vi "PulseLengthen.vi"(7 "Lengthen":u32, 10 "Pulse":bool) -> (2 "Lengthened":bool)   [LabVIEW 2014]
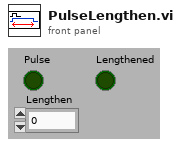
[diagram p1: front panel]
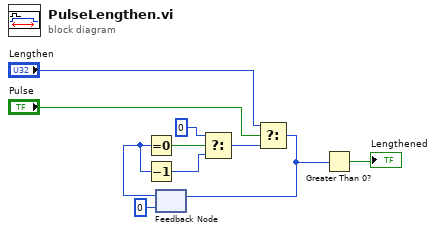
[diagram p0: block diagram]
diagram:
  n1 = feedback #1(u32 0 ("t")) -> (w2:u32)
  n2 = Equal To 0?(x=w2) -> (x = 0?=w7:bool)
  n3 = Decrement(x=w2) -> (x-1=w4:u32)
  n4 = Select(t=u32 0, s=w7, f=w4) -> (s? t:f=w5:u32)
  n5 = Select(t="Lengthen", s="Pulse", f=w5) -> (s? t:f=w3:u32)
  n6 = feedback-in #1(w3) -> ()
  n7 = Greater Than 0?(x=w3) -> (x > 0?=→"Lengthened":bool)
